vi "Set Reference Range COM Port.vi"(8 "error in (no error)":errorcluster, 10 "Reference Range COM Port":refnum<visa-resource-name>, 11 "Reference Range Actor in":refnum<class "Reference Range Actor.lvclass">) -> (0 "error out":errorcluster, 3 "Reference Range Actor out":refnum<class "Reference Range Actor.lvclass">)   [LabVIEW 2017]
uses:
  Reference Range Actor.lvclass
  C:/Users/dev/Documents/CODE/LabVIEW/microwaveverify/trunk/MWWL Verification/Actor Monitor/Actor/Monitored Actor.lvclass
  C:/Program Files (x86)/National Instruments/LabVIEW 2017/vi.lib/ActorFramework/Actor/Actor.lvclass
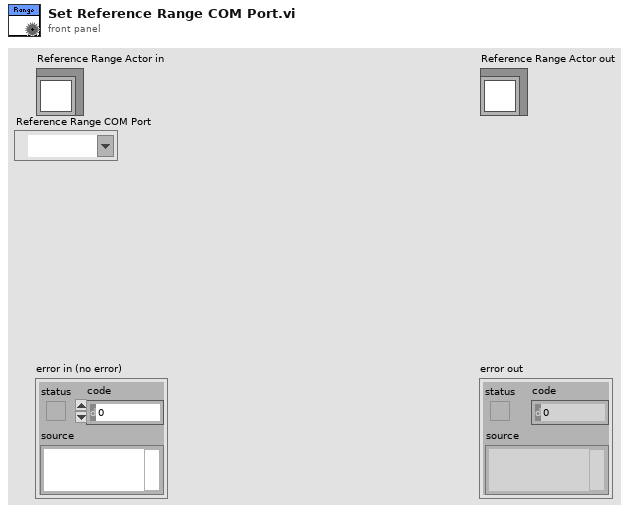
[diagram p1: front panel]
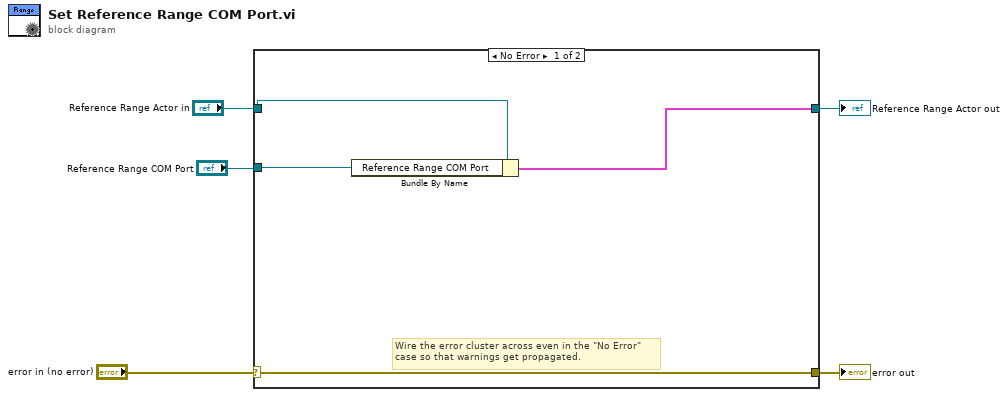
[diagram p0: block diagram]
diagram:
  n1 = case shown="No Error" "error in (no error)" {
    selector: "error in (no error)" -> [w9 w11]
    tunnel: [w9 w11] -> w4
    tunnel: [w7 w10] -> w2
    tunnel: "Reference Range Actor in" -> [w8 w10]
    tunnel: "Reference Range COM Port" -> [w6 _]
    frame No Error {
      # "Wire the error cluster across even in the \"No Error\"\ncase so that warnings get propagated."
      n2 = Bundle By Name(cluster=w8, "Reference Range COM Port"=w6) -> (w7:cluster{})
    }
    frame Error {
    }
  }
  "error out" <- w4
  "Reference Range Actor out" <- w2
